vi "Car Wash Controller.vi"(8 "error in (no error)":errorcluster, 11 "Message Queues":T1) -> (0 "error out":errorcluster)   [LabVIEW 2017]
uses:
  support/Message Queue/All Message Queues.ctl
  support/Message Queue/Message Cluster.ctl
  Position Slider.ctl
  Entry Display Data.ctl
  Wash Step Indicators.ctl
  support/Message Queue/Enqueue Message (Single).vi
  <vilib>/ErrorRing/Error Ring.xnode
  support/Message Queue/Message Queue.lvlib
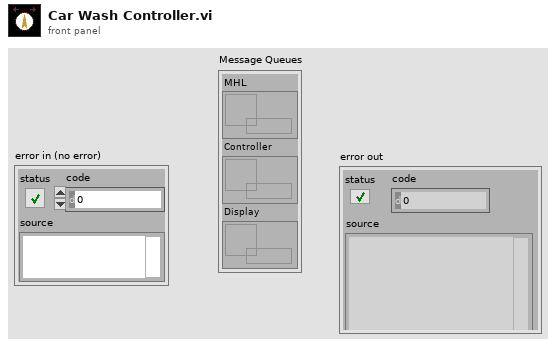
[diagram p1: front panel]
types:
  T1 = typedef "Message Queue.lvlib/All Message Queues.ctl" = cluster{"MHL":refnum<queue>, "Controller":refnum<queue>, "Display":refnum<queue>}
  T2 = enum16{"Entry", "Under Body Wash", "Bug Remover", "Pre-Soak", "High Pressure Wash", "Low Pressure Wax", "Spot Free Rinse", "Tire Shine Foam", "Air Dry", "Exit"}
  T3 = typedef "Position Slider.ctl" = i32
  T4 = typedef "Entry Display Data.ctl" = cluster{"Wash Entry Display":bool, "Car Position Slider":T3, "Wash Display Indicators":T5, "Vehicle Postion":bool}
  T5 = typedef "Wash Step Indicators.ctl" = cluster{"Under Body Wash":bool, "Bug Remover":bool, "Pre-soak":bool, " High Pressure Wash":bool, "Low Pressure  Wax":bool, "Spot Free Rinse":bool, " Tire Shine Foam":bool, " Air Dry":bool}
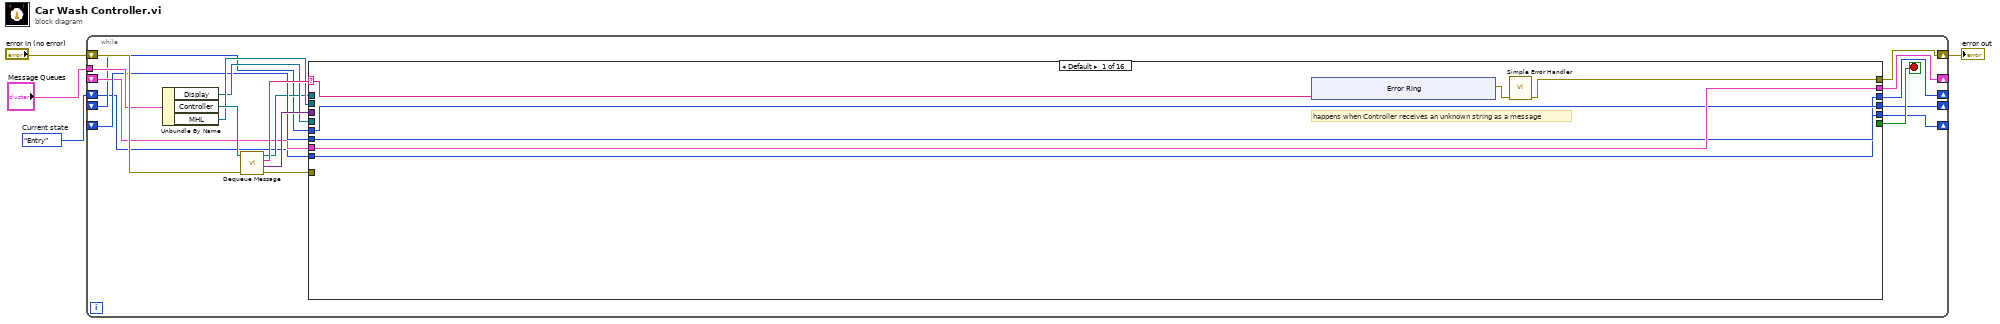
[diagram p0: block diagram]
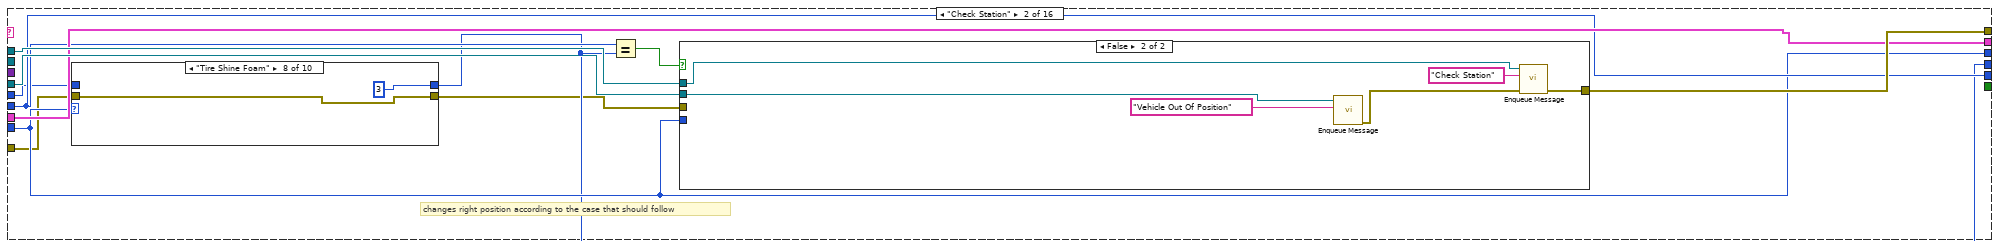
[diagram p2: hidden frame]
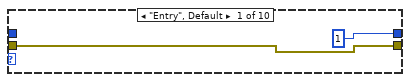
[diagram p3: hidden frame]
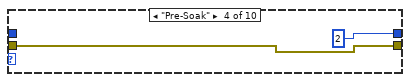
[diagram p6: hidden frame]
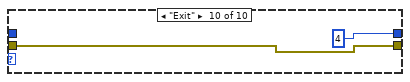
[diagram p11: hidden frame]
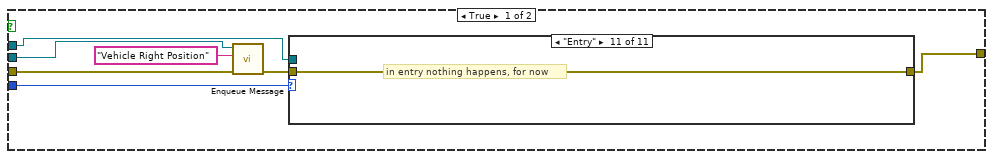
[diagram p12: hidden frame]
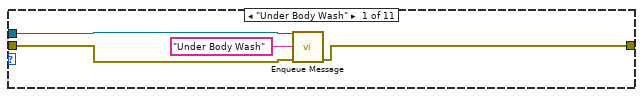
[diagram p13: hidden frame]
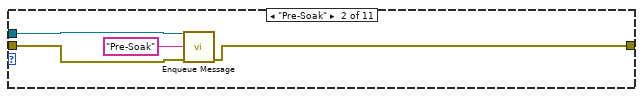
[diagram p14: hidden frame]
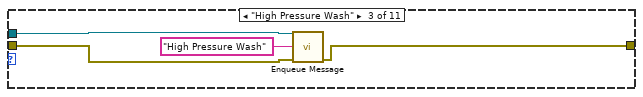
[diagram p15: hidden frame]
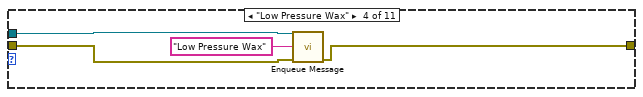
[diagram p16: hidden frame]
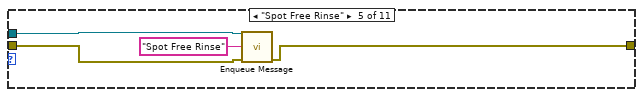
[diagram p17: hidden frame]
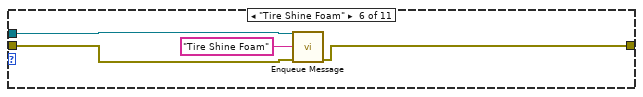
[diagram p18: hidden frame]
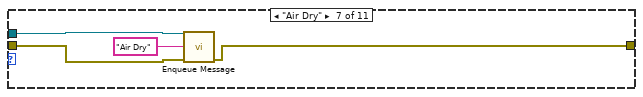
[diagram p19: hidden frame]
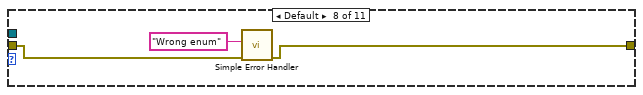
[diagram p20: hidden frame]
diagram:
  w1 = T2."Entry"  # Current state
  n1 = while {
    shift-right: [w18] -> w3
    shift-left: "error in (no error)" -> [w23]
    shift-right: [w19] -> _
    shift-left: _ -> [w9]
    tunnel: "Message Queues" -> [w16]
    shift-right: [w12] -> _
    shift-left: _ -> [w11]
    shift-right: [w8] -> _
    shift-left: _ -> [w7]
    shift-right: [w6] -> _
    shift-left: w1 -> [w5]
    stop <- w17 stop-if-true
    n2 = Unbundle By Name(w16) -> ("Display"=w13:refnum<queue>, "Controller"=w20:refnum<queue>, "MHL"=w14:refnum<queue>)
    n3 = call "Dequeue Message.vi"("error in (no error)"=w23, "Message Queue"=w20) -> ("error out"=w21:errorcluster, "Message Data"=w22:variant, "Message"=w15:string, "dup Message Queue"=w10:refnum<queue>)  [unwired: 6 in]
    n4 = case shown="Default" w15 {
      selector: w15 -> [w30 _ _ _ _ _ _ _ _ _ _ _ _ _ _ _]
      tunnel: w22 -> [_ _ _ _ _ _ w197 w209 _ _ _ _ _ _ _ _]
      tunnel: w21 -> [_ w37 w121 _ w169 w182 w196 w202 w217 w244 w275 w306 w337 w365 w393 w421]
      tunnel: [w29 w42 w124 w138 w172 w185 w194 w207 w213 w241 w271 w302 w331 w361 w389 w415] -> w19
      tunnel: w9 -> [w29 w42 w124 w138 w172 w185 w194 _ w213 w241 w271 w302 w331 w361 w389 w415]
      tunnel: [w27 w44 w121 w126 w168 w177 w187 w205 w215 w238 w273 w304 w335 w363 w391 w419] -> w18
      tunnel: [_ _ _ _ _ TRUE FALSE _ _ _ _ _ _ _ _ _] -> w17
      tunnel: w14 -> [_ _ _ _ _ w174 _ _ _ _ _ _ _ _ _ _]
      tunnel: w13 -> [_ w45 _ w136 w171 w181 _ _ w218 w242 w272 w303 w334 w362 w390 w418]
      tunnel: [w26 w41 w123 w130 w167 w176 w191 w204 w219 w245 w276 w307 w338 w366 w394 w422] -> w12
      tunnel: w11 -> [w26 w41 w123 w130 w167 w176 _ w204 w219 w245 w276 w307 w338 w366 w394 w422]
      tunnel: w10 -> [_ w43 _ w137 _ _ w189 _ w216 w243 w274 w305 w336 w364 w392 w420]
      tunnel: [w25 w38 w122 w125 w166 w175 w192 1 ("Right Position") w214 w239 w269 w300 w332 w359 w387 w416] -> w8
      tunnel: w7 -> [w25 w39 w122 w125 _ w175 w192 _ w214 w240 w270 w301 w333 w360 w388 w417]
      tunnel: w5 -> [w24 w40 w120 w131 w165 w173 w186 _ w211 w236 w267 w298 w329 w357 w385 w413]
      tunnel: [w24 w40 w120 w127 w165 w173 w186 w198 w210 w235 w266 w297 w328 w356 w384 w412] -> w6
      frame Default {
        # "happens when Controller receives an unknown string as a message"
        n5 = xnode "Error Ring"("parameter 0"=w30) -> ("error out"=w28:errorcluster)
        n6 = call <vilib>:"Simple Error Handler.vi"("error in (no error)"=w28) -> ("error out"=w27:errorcluster)  [unwired: 4 in, 4 out]
      }
      frame "Check Station" {
        # "changes right position according to the case that should follow"
        n7 = case shown="\"Tire Shine Foam\"" w40 {
          tunnel: w39 -> [_ w50 w52 _ w56 w58 w60 _ w64 _]
          tunnel: [1 ("Right Position") w50 w52 2 ("Right Position") w56 w58 w60 3 ("Right Position") w64 4 ("Right Position")] -> w38
          tunnel: w37 -> [w47 w49 w51 w53 w55 w57 w59 w61 w63 w65]
          tunnel: [w47 w49 w51 w53 w55 w57 w59 w61 w63 w65] -> w36
          frame "Entry", Default {
          }
          frame "Under Body Wash" {
          }
          frame "Bug Remover" {
          }
          frame "Pre-Soak" {
          }
          frame "High Pressure Wash" {
          }
          frame "Low Pressure Wax" {
          }
          frame "Spot Free Rinse" {
          }
          frame "Tire Shine Foam" {
          }
          frame "Air Dry" {
          }
          frame "Exit" {
          }
        }
        n8 = Equal?(x=w41, y=w38) -> (x = y?=w46:bool)
        n9 = case shown="False" w46 {
          tunnel: w45 -> [w73 w118]
          tunnel: [w68 w114] -> w44
          tunnel: w43 -> [w70 w117]
          tunnel: w40 -> [w71 _]
          tunnel: w36 -> [w67 _]
          frame True {
            n10 = call-poly "Enqueue Message.vi"("error in (no error)"=w67, "Message"="Vehicle Right Position", "Message Queue"=w73) -> ("error out"=w69:errorcluster)  [unwired: 7 in, 1 out]
            n11 = case shown="\"Entry\"" w71 {
              tunnel: w69 -> [w76 w80 w84 w88 w92 w96 w100 w104 w107 w111 w113]
              tunnel: [w75 w79 w83 w87 w91 w95 w99 w103 w106 w110 w113] -> w68
              tunnel: w70 -> [w74 w78 w82 w86 w90 w94 w98 _ w105 w112 _]
              frame "Under Body Wash" {
                n12 = call-poly "Enqueue Message.vi"("error in (no error)"=w76, "Message"="Under Body Wash", "Message Queue"=w74) -> ("error out"=w75:errorcluster)  [unwired: 7 in, 1 out]
              }
              frame "Pre-Soak" {
                n13 = call-poly "Enqueue Message.vi"("error in (no error)"=w80, "Message"="Pre-Soak", "Message Queue"=w78) -> ("error out"=w79:errorcluster)  [unwired: 7 in, 1 out]
              }
              frame "High Pressure Wash" {
                n14 = call-poly "Enqueue Message.vi"("error in (no error)"=w84, "Message"="High Pressure Wash", "Message Queue"=w82) -> ("error out"=w83:errorcluster)  [unwired: 7 in, 1 out]
              }
              frame "Low Pressure Wax" {
                n15 = call-poly "Enqueue Message.vi"("error in (no error)"=w88, "Message"="Low Pressure Wax", "Message Queue"=w86) -> ("error out"=w87:errorcluster)  [unwired: 7 in, 1 out]
              }
              frame "Spot Free Rinse" {
                n16 = call-poly "Enqueue Message.vi"("error in (no error)"=w92, "Message"="Spot Free Rinse", "Message Queue"=w90) -> ("error out"=w91:errorcluster)  [unwired: 7 in, 1 out]
              }
              frame "Tire Shine Foam" {
                n17 = call-poly "Enqueue Message.vi"("error in (no error)"=w96, "Message"="Tire Shine Foam", "Message Queue"=w94) -> ("error out"=w95:errorcluster)  [unwired: 7 in, 1 out]
              }
              frame "Air Dry" {
                n18 = call-poly "Enqueue Message.vi"("error in (no error)"=w100, "Message"="Air Dry", "Message Queue"=w98) -> ("error out"=w99:errorcluster)  [unwired: 7 in, 1 out]
              }
              frame Default {
                n19 = call <vilib>:"Simple Error Handler.vi"("error source (\" \")"="Wrong enum" ("error source (\" \")"), "error in (no error)"=w104) -> ("error out"=w103:errorcluster)  [unwired: 3 in, 4 out]
              }
              frame "Bug Remover" {
                n20 = call-poly "Enqueue Message.vi"("error in (no error)"=w107, "Message"="Bug Remover", "Message Queue"=w105) -> ("error out"=w106:errorcluster)  [unwired: 7 in, 1 out]
              }
              frame "Exit" {
                n21 = call-poly "Enqueue Message.vi"("error in (no error)"=w111, "Message"="Exit", "Message Queue"=w112) -> ("error out"=w110:errorcluster)  [unwired: 7 in, 1 out]
              }
              frame "Entry" {
                # "in entry nothing happens, for now"
              }
            }
          }
          frame False {
            n22 = call-poly "Enqueue Message.vi"("Message"="Vehicle Out Of Position", "Message Queue"=w118) -> ("error out"=w116:errorcluster)  [unwired: 8 in, 1 out]
            n23 = call-poly "Enqueue Message.vi"("error in (no error)"=w116, "Message"="Check Station", "Message Queue"=w117) -> ("error out"=w114:errorcluster)  [unwired: 7 in, 1 out]
          }
        }
      }
      frame "Entry" {
      }
      frame "Check time" {
        w134 = 5.0 ("Time Limit")
        # "pauses if the car is not in the expected position"
        n24 = Equal?(x=w125, y=w130) -> (x = y?=w129:bool)
        n25 = Not(x=w129) -> (.not. x?=w128:bool)
        n26 = call "Timer.vi"("Time Limit"=w134, "Pause"=w128) -> ("error out"=w135:errorcluster, "Elapsed Time"=w133:dbl, "Time Expired?"=w132:bool)  [unwired: 7 in]
        n27 = case shown="True" w132 {
          tunnel: w137 -> [w149 w150]
          tunnel: [w141 w162] -> w126
          tunnel: w136 -> [w143 w159]
          tunnel: w135 -> [w147 w154]
          tunnel: w134 -> [w146 _]
          tunnel: w133 -> [w145 _]
          tunnel: w131 -> [w139 w152]
          tunnel: [w139 w151] -> w127
          frame False {
            # "recursively enter the check time case"
            # "update time indicator"
            n28 = Subtract(x=w146, y=w145) -> (x-y=w144:dbl)
            n29 = call-poly "Enqueue Message.vi"("error in (no error)"=w147, "Message"="Check time", "Message Queue"=w149) -> ("error out"=w140:errorcluster)  [unwired: 7 in, 1 out]
            n30 = call-poly "Enqueue Message.vi"("error in (no error)"=w140, "Message Data"=w144, "Message"="Time Remaining", "Message Queue"=w143) -> ("error out"=w141:errorcluster)  [unwired: 6 in, 1 out]
          }
          frame True {
            n31 = call "Timer.vi"("error in"=w154, "Time Limit"=2.0, "Reset"=TRUE) -> ("error out"=w155:errorcluster, "Elapsed Time"=w153:dbl)  [unwired: 6 in, 1 out]
            n32 = call-poly "Enqueue Message.vi"("error in (no error)"=w155, "Message Data"=w153, "Message"="Time Remaining", "Message Queue"=w159) -> ("error out"=w156:errorcluster)  [unwired: 6 in, 1 out]
            n33 = call-poly "Enqueue Message.vi"("error in (no error)"=w156, "Message"="Indicators Off", "Message Queue"=w159) -> ("error out"=w161:errorcluster)  [unwired: 7 in, 1 out]
            n34 = call-poly "Enqueue Message.vi"("error in (no error)"=w161, "Message"="Check Station", "Message Queue"=w150) -> ("error out"=w162:errorcluster)  [unwired: 7 in, 1 out]
            n35 = Increment(x=w152) -> (x+1=w151:T2)
          }
        }
      }
      frame "Initialize" {
        w166 = 0  # Right Position
        # "wash display indicators are all off on init"
        n36 = call-poly "Enqueue Message.vi"("error in (no error)"=w169, "Message"="Indicators Off", "Message Queue"=w171) -> ("error out"=w168:errorcluster)  [unwired: 7 in, 1 out]
      }
      frame "Exit" {
        # "controls are all off and clickable again on exit station"
        n37 = call-poly "Enqueue Message.vi"("Message"="Wash Vacant", "Message Queue"=w181) -> ("error out"=w179:errorcluster)  [unwired: 8 in, 1 out]
        n38 = call-poly "Enqueue Message.vi"("error in (no error)"=w182, "Message"="Restore Controls", "Message Queue"=w174) -> ("error out"=w178:errorcluster)  [unwired: 7 in, 1 out]
        n39 = Merge Errors(w179, w178) -> (w177:errorcluster)
      }
      frame "Change Station" {
        n40 = Variant To Data(error in=w196, type=T3 0 ("Car Position Slider"), Variant=w197) -> (data=w191:T3, error out=w190:errorcluster)
        n41 = call-poly "Enqueue Message.vi"("error in (no error)"=w190, "Message"="Check Station", "Message Queue"=w189) -> ("error out"=w187:errorcluster)  [unwired: 7 in, 1 out]
      }
      frame "Start Wash" {
        w198 = T2."Under Body Wash"  # Current state
        n42 = One Button Dialog(message="Start Wash") -> ()  [unwired: 1 in, 1 out]
        n43 = call "Timer.vi"("error in"=w202, "Time Limit"=5.0, "Reset"=TRUE) -> ("error out"=w201:errorcluster)  [unwired: 6 in, 2 out]
        n44 = Variant To Data(error in=w201, type=T4 {"Wash Entry Display"=FALSE, "Car Position Slider"=0, "Wash Display Indicators"={"Under Body Wash"=FALSE, "Bug Remover"=FALSE, "Pre-soak"=FALSE, " High Pressure Wash"=FALSE, "Low Pressure  Wax"=FALSE, "Spot Free Rinse"=FALSE, " Tire Shine Foam"=FALSE, " Air Dry"=FALSE}, "Vehicle Postion"=FALSE} ("Cluster"), Variant=w209) -> (data=w207:T4, error out=w205:errorcluster)
      }
      frame "Under Body Wash" {
        n45 = Unbundle By Name(w213) -> ("Wash Display Indicators.Under Body Wash"=w212:bool)
        n46 = case shown="False" w212 {
          tunnel: w218 -> [_ w234]
          tunnel: w217 -> [w223 w227]
          tunnel: w216 -> [w225 w232]
          tunnel: [w222 w231] -> w215
          tunnel: w211 -> [w221 w226]
          tunnel: [w220 w226] -> w210
          frame False {
            # "always check station before the next state to check the vehicle position and set the right expected station!!"
            # "if the state isn't required, current state changes to the next state"
            n47 = Increment(x=w221) -> (x+1=w220:T2)
            n48 = call-poly "Enqueue Message.vi"("error in (no error)"=w223, "Message"="Check Station", "Message Queue"=w225) -> ("error out"=w222:errorcluster)  [unwired: 7 in, 1 out]
          }
          frame True {
            # "light the indicator"
            n49 = call-poly "Enqueue Message.vi"("error in (no error)"=w227, "Message Data"=T5 {"Under Body Wash"=TRUE, "Bug Remover"=FALSE, "Pre-soak"=FALSE, " High Pressure Wash"=FALSE, "Low Pressure  Wax"=FALSE, "Spot Free Rinse"=FALSE, " Tire Shine Foam"=FALSE, " Air Dry"=FALSE} ("Wash Step Indicators"), "Message"="Update Interface", "Message Queue"=w234) -> ("error out"=w228:errorcluster)  [unwired: 6 in, 1 out]
            n50 = call-poly "Enqueue Message.vi"("error in (no error)"=w228, "Message"="Check time", "Message Queue"=w232) -> ("error out"=w231:errorcluster)  [unwired: 7 in, 1 out]
          }
        }
      }
      frame "Bug Remover" {
        # "if this state was selected & if it hasn't been lit before"
        n51 = Unbundle By Name(w241) -> ("Wash Display Indicators.Bug Remover"=w237:bool)
        n52 = case shown="False" w237 {
          tunnel: w242 -> [_ w265]
          tunnel: w244 -> [w253 w264]
          tunnel: w243 -> [w255 w262]
          tunnel: [w249 w260] -> w238
          tunnel: w242 -> [w252 _]
          tunnel: w240 -> [w248 w258]
          tunnel: [w248 w258] -> w239
          tunnel: w236 -> [w247 w256]
          tunnel: [w246 w256] -> w235
          frame False {
            # "always check station before the next state to check the vehicle position and set the right expected station!!"
            # "if the state isn't required, current state changes to the next state"
            n53 = Increment(x=w247) -> (x+1=w246:T2)
            n54 = call-poly "Enqueue Message.vi"("error in (no error)"=w253, "Message"="Check Station", "Message Queue"=w255) -> ("error out"=w250:errorcluster)  [unwired: 7 in, 1 out]
            n55 = call-poly "Enqueue Message.vi"("error in (no error)"=w250, "Message"="Vehicle Out Of Position", "Message Queue"=w252) -> ("error out"=w249:errorcluster)  [unwired: 7 in, 1 out]
          }
          frame True {
            n56 = call-poly "Enqueue Message.vi"("error in (no error)"=w264, "Message Data"=T5 {"Under Body Wash"=FALSE, "Bug Remover"=TRUE, "Pre-soak"=FALSE, " High Pressure Wash"=FALSE, "Low Pressure  Wax"=FALSE, "Spot Free Rinse"=FALSE, " Tire Shine Foam"=FALSE, " Air Dry"=FALSE} ("Wash Step Indicators"), "Message"="Update Interface", "Message Queue"=w265) -> ("error out"=w257:errorcluster)  [unwired: 6 in, 1 out]
            n57 = call-poly "Enqueue Message.vi"("error in (no error)"=w257, "Message"="Check time", "Message Queue"=w262) -> ("error out"=w260:errorcluster)  [unwired: 7 in, 1 out]
          }
        }
      }
      frame "Spot Free Rinse" {
        # "if this state was selected & if it hasn't been lit before"
        n58 = Unbundle By Name(w271) -> ("Wash Display Indicators.Spot Free Rinse"=w268:bool)
        n59 = case shown="False" w268 {
          tunnel: w272 -> [_ w296]
          tunnel: w275 -> [w284 w295]
          tunnel: w274 -> [w286 w293]
          tunnel: [w280 w291] -> w273
          tunnel: w272 -> [w283 _]
          tunnel: w270 -> [w279 w289]
          tunnel: [w279 w289] -> w269
          tunnel: w267 -> [w277 w287]
          tunnel: [w278 w287] -> w266
          frame False {
            # "always check station before the next state to check the vehicle position and set the right expected station!!"
            # "if the state isn't required, current state changes to the next state"
            n60 = Increment(x=w277) -> (x+1=w278:T2)
            n61 = call-poly "Enqueue Message.vi"("error in (no error)"=w284, "Message"="Check Station", "Message Queue"=w286) -> ("error out"=w281:errorcluster)  [unwired: 7 in, 1 out]
            n62 = call-poly "Enqueue Message.vi"("error in (no error)"=w281, "Message"="Vehicle Out Of Position", "Message Queue"=w283) -> ("error out"=w280:errorcluster)  [unwired: 7 in, 1 out]
          }
          frame True {
            n63 = call-poly "Enqueue Message.vi"("error in (no error)"=w295, "Message Data"=T5 {"Under Body Wash"=FALSE, "Bug Remover"=FALSE, "Pre-soak"=FALSE, " High Pressure Wash"=FALSE, "Low Pressure  Wax"=FALSE, "Spot Free Rinse"=TRUE, " Tire Shine Foam"=FALSE, " Air Dry"=FALSE} ("Wash Step Indicators"), "Message"="Update Interface", "Message Queue"=w296) -> ("error out"=w288:errorcluster)  [unwired: 6 in, 1 out]
            n64 = call-poly "Enqueue Message.vi"("error in (no error)"=w288, "Message"="Check time", "Message Queue"=w293) -> ("error out"=w291:errorcluster)  [unwired: 7 in, 1 out]
          }
        }
      }
      frame "Air Dry" {
        # "if this state was selected & if it hasn't been lit before"
        n65 = Unbundle By Name(w302) -> ("Wash Display Indicators.Air Dry"=w299:bool)
        n66 = case shown="False" w299 {
          tunnel: w303 -> [_ w327]
          tunnel: w306 -> [w315 w326]
          tunnel: w305 -> [w317 w324]
          tunnel: [w311 w322] -> w304
          tunnel: w303 -> [w314 _]
          tunnel: w301 -> [w310 w320]
          tunnel: [w310 w320] -> w300
          tunnel: w298 -> [w309 w318]
          tunnel: [w308 w318] -> w297
          frame False {
            # "always check station before the next state to check the vehicle position and set the right expected station!!"
            # "if the state isn't required, current state changes to the next state"
            n67 = Increment(x=w309) -> (x+1=w308:T2)
            n68 = call-poly "Enqueue Message.vi"("error in (no error)"=w315, "Message"="Check Station", "Message Queue"=w317) -> ("error out"=w312:errorcluster)  [unwired: 7 in, 1 out]
            n69 = call-poly "Enqueue Message.vi"("error in (no error)"=w312, "Message"="Vehicle Out Of Position", "Message Queue"=w314) -> ("error out"=w311:errorcluster)  [unwired: 7 in, 1 out]
          }
          frame True {
            n70 = call-poly "Enqueue Message.vi"("error in (no error)"=w326, "Message Data"=T5 {"Under Body Wash"=FALSE, "Bug Remover"=FALSE, "Pre-soak"=FALSE, " High Pressure Wash"=FALSE, "Low Pressure  Wax"=FALSE, "Spot Free Rinse"=FALSE, " Tire Shine Foam"=FALSE, " Air Dry"=TRUE} ("Wash Step Indicators"), "Message"="Update Interface", "Message Queue"=w327) -> ("error out"=w319:errorcluster)  [unwired: 6 in, 1 out]
            n71 = call-poly "Enqueue Message.vi"("error in (no error)"=w319, "Message"="Check time", "Message Queue"=w324) -> ("error out"=w322:errorcluster)  [unwired: 7 in, 1 out]
          }
        }
      }
      frame "Tire Shine Foam" {
        n72 = Unbundle By Name(w331) -> ("Wash Display Indicators.Tire Shine Foam"=w330:bool)
        n73 = case shown="False" w330 {
          tunnel: w334 -> [_ w355]
          tunnel: w337 -> [w343 w354]
          tunnel: w336 -> [w345 w352]
          tunnel: [w341 w350] -> w335
          tunnel: w334 -> [_ _]
          tunnel: w333 -> [w342 w348]
          tunnel: [w342 w348] -> w332
          tunnel: w329 -> [w340 w346]
          tunnel: [w339 w346] -> w328
          frame False {
            # "always check station before the next state to check the vehicle position and set the right expected station!!"
            # "if the state isn't required, current state changes to the next state"
            n74 = Increment(x=w340) -> (x+1=w339:T2)
            n75 = call-poly "Enqueue Message.vi"("error in (no error)"=w343, "Message"="Check Station", "Message Queue"=w345) -> ("error out"=w341:errorcluster)  [unwired: 7 in, 1 out]
          }
          frame True {
            n76 = call-poly "Enqueue Message.vi"("error in (no error)"=w354, "Message Data"=T5 {"Under Body Wash"=FALSE, "Bug Remover"=FALSE, "Pre-soak"=FALSE, " High Pressure Wash"=FALSE, "Low Pressure  Wax"=FALSE, "Spot Free Rinse"=FALSE, " Tire Shine Foam"=TRUE, " Air Dry"=FALSE} ("Wash Step Indicators"), "Message"="Update Interface", "Message Queue"=w355) -> ("error out"=w347:errorcluster)  [unwired: 6 in, 1 out]
            n77 = call-poly "Enqueue Message.vi"("error in (no error)"=w347, "Message"="Check time", "Message Queue"=w352) -> ("error out"=w350:errorcluster)  [unwired: 7 in, 1 out]
          }
        }
      }
      frame "Low Pressure Wax" {
        # "if this state was selected & if it hasn't been lit before"
        n78 = Unbundle By Name(w361) -> ("Wash Display Indicators.Low Pressure  Wax"=w358:bool)
        n79 = case shown="True" w358 {
          tunnel: w362 -> [_ w383]
          tunnel: w365 -> [w371 w382]
          tunnel: w364 -> [w373 w376]
          tunnel: [w370 w379] -> w363
          tunnel: w362 -> [_ _]
          tunnel: w360 -> [w369 w377]
          tunnel: [w369 w377] -> w359
          tunnel: w357 -> [w368 w374]
          tunnel: [w367 w374] -> w356
          frame False {
            # "always check station before the next state to check the vehicle position and set the right expected station!!"
            # "if the state isn't required, current state changes to the next state"
            n80 = Increment(x=w368) -> (x+1=w367:T2)
            n81 = call-poly "Enqueue Message.vi"("error in (no error)"=w371, "Message"="Check Station", "Message Queue"=w373) -> ("error out"=w370:errorcluster)  [unwired: 7 in, 1 out]
          }
          frame True {
            n82 = call-poly "Enqueue Message.vi"("error in (no error)"=w382, "Message Data"=T5 {"Under Body Wash"=FALSE, "Bug Remover"=FALSE, "Pre-soak"=FALSE, " High Pressure Wash"=FALSE, "Low Pressure  Wax"=TRUE, "Spot Free Rinse"=FALSE, " Tire Shine Foam"=FALSE, " Air Dry"=FALSE} ("Wash Step Indicators"), "Message"="Update Interface", "Message Queue"=w383) -> ("error out"=w375:errorcluster)  [unwired: 6 in, 1 out]
            n83 = call-poly "Enqueue Message.vi"("error in (no error)"=w375, "Message"="Check time", "Message Queue"=w376) -> ("error out"=w379:errorcluster)  [unwired: 7 in, 1 out]
          }
        }
      }
      frame "Pre-Soak" {
        # "if this state was selected & if it hasn't been lit before"
        n84 = Unbundle By Name(w389) -> ("Wash Display Indicators.Pre-soak"=w386:bool)
        n85 = case shown="False" w386 {
          tunnel: w390 -> [_ w411]
          tunnel: w393 -> [w399 w410]
          tunnel: w392 -> [w401 w408]
          tunnel: [w398 w406] -> w391
          tunnel: w390 -> [_ _]
          tunnel: w388 -> [w397 w404]
          tunnel: [w397 w404] -> w387
          tunnel: w385 -> [w396 w402]
          tunnel: [w395 w402] -> w384
          frame False {
            # "always check station before the next state to check the vehicle position and set the right expected station!!"
            # "if the state isn't required, current state changes to the next state"
            n86 = Increment(x=w396) -> (x+1=w395:T2)
            n87 = call-poly "Enqueue Message.vi"("error in (no error)"=w399, "Message"="Check Station", "Message Queue"=w401) -> ("error out"=w398:errorcluster)  [unwired: 7 in, 1 out]
          }
          frame True {
            n88 = call-poly "Enqueue Message.vi"("error in (no error)"=w410, "Message Data"=T5 {"Under Body Wash"=FALSE, "Bug Remover"=FALSE, "Pre-soak"=TRUE, " High Pressure Wash"=FALSE, "Low Pressure  Wax"=FALSE, "Spot Free Rinse"=FALSE, " Tire Shine Foam"=FALSE, " Air Dry"=FALSE} ("Wash Step Indicators"), "Message"="Update Interface", "Message Queue"=w411) -> ("error out"=w403:errorcluster)  [unwired: 6 in, 1 out]
            n89 = call-poly "Enqueue Message.vi"("error in (no error)"=w403, "Message"="Check time", "Message Queue"=w408) -> ("error out"=w406:errorcluster)  [unwired: 7 in, 1 out]
          }
        }
      }
      frame "High Pressure Wash" {
        n90 = Unbundle By Name(w415) -> ("Wash Display Indicators.High Pressure Wash"=w414:bool)
        n91 = case shown="False" w414 {
          tunnel: w418 -> [_ w439]
          tunnel: w421 -> [w427 w438]
          tunnel: w420 -> [w429 w436]
          tunnel: [w426 w434] -> w419
          tunnel: w418 -> [_ _]
          tunnel: w417 -> [w425 w432]
          tunnel: [w425 w432] -> w416
          tunnel: [w424 w430] -> w412
          tunnel: w413 -> [w423 w430]
          frame False {
            # "always check station before the next state to check the vehicle position and set the right expected station!!"
            # "if the state isn't required, current state changes to the next state"
            n92 = Increment(x=w423) -> (x+1=w424:T2)
            n93 = call-poly "Enqueue Message.vi"("error in (no error)"=w427, "Message"="Check Station", "Message Queue"=w429) -> ("error out"=w426:errorcluster)  [unwired: 7 in, 1 out]
          }
          frame True {
            n94 = call-poly "Enqueue Message.vi"("error in (no error)"=w438, "Message Data"=T5 {"Under Body Wash"=FALSE, "Bug Remover"=FALSE, "Pre-soak"=FALSE, " High Pressure Wash"=TRUE, "Low Pressure  Wax"=FALSE, "Spot Free Rinse"=FALSE, " Tire Shine Foam"=FALSE, " Air Dry"=FALSE} ("Wash Step Indicators"), "Message"="Update Interface", "Message Queue"=w439) -> ("error out"=w431:errorcluster)  [unwired: 6 in, 1 out]
            n95 = call-poly "Enqueue Message.vi"("error in (no error)"=w431, "Message"="Check time", "Message Queue"=w436) -> ("error out"=w434:errorcluster)  [unwired: 7 in, 1 out]
          }
        }
      }
    }
  }
  "error out" <- w3
